vi "Set Node IDs.vi"(8 "error in":errorcluster, 9 "Tester Tx":refnum<vi>, 10 "Tester Rx":refnum<vi>, 11 "PLC Controller in":refnum<class "PLC Sim Controller Actor.lvclass">) -> (0 "error out":errorcluster, 3 "PLC Controller out":refnum<class "PLC Sim Controller Actor.lvclass">)   [LabVIEW 2019]
uses:
  PLC Sim Controller Actor.lvclass
  C:/Program Files (x86)/National Instruments/LabVIEW 2019/vi.lib/ActorFramework/Actor/Actor.lvclass
  <vilib>/ActorFramework/Message Enqueuer/Message Enqueuer.lvclass
  Station Actor/Station Actor/Custom Controls/Tester Rx Dataset.ctl
  Station Actor/Station Actor/Station Actor.lvclass
  Station Actor/Station Actor/Custom Controls/Tester Tx Dataset.ctl
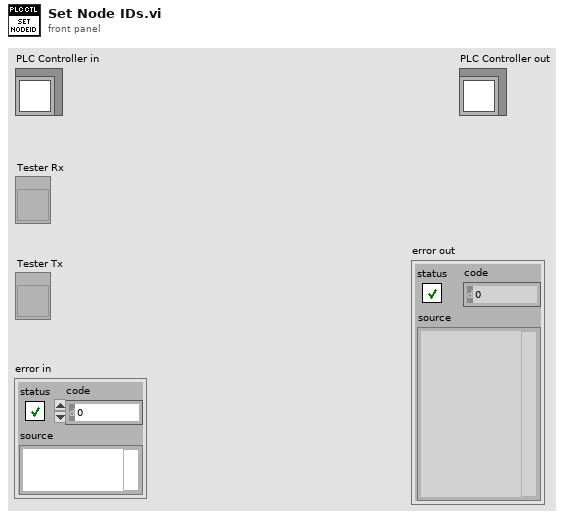
[diagram p1: front panel]
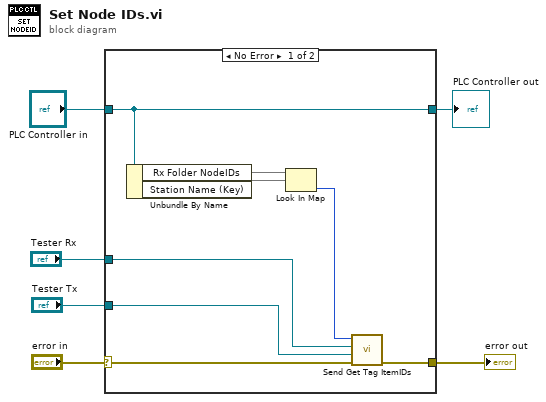
[diagram p0: block diagram]
diagram:
  n1 = case shown="No Error" "error in" {
    selector: "error in" -> [w12 w15]
    tunnel: "PLC Controller in" -> [w10 w16]
    tunnel: [w10 w16] -> w4
    tunnel: [w11 w15] -> w3
    tunnel: "Tester Rx" -> [w14 _]
    tunnel: "Tester Tx" -> [w13 _]
    frame No Error {
      n2 = Unbundle By Name(w10) -> ("Rx Folder NodeIDs"=w9, "Station Name (Key)"=w7)
      n3 = Look In Map(map=w9, key=w7) -> (value=w8:i32)  [unwired: 1 in, 1 out]
      n4 = call "Send Get Tag ItemIDs.vi"("error in (no error)"=w12, "Tester Tx"=w13, "Tester Rx"=w14, "Message Enqueuer"=w8) -> ("error out"=w11:errorcluster)  [unwired: 6 in, 1 out]
    }
    frame Error {
    }
  }
  "error out" <- w3
  "PLC Controller out" <- w4
